vi "Four 64 bit to 256 bit pack.vi"(6 "Flush?":bool, 8 "Input Valid":bool, 11 "Input Data":u64) -> (0 "Output Valid":bool, 3 "Output Data":T1)   [LabVIEW 2011]
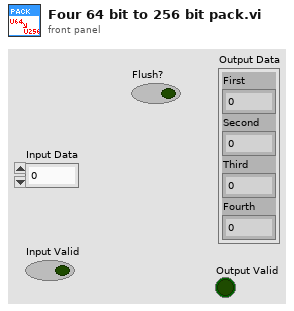
[diagram p1: front panel]
types:
  T1 = cluster{"First":u64, "Second":u64, "Third":u64, "Fourth":u64}
  T2 = cluster{"[0]":u64, "[1]":u64, "[2]":u64, "[3]":u64}
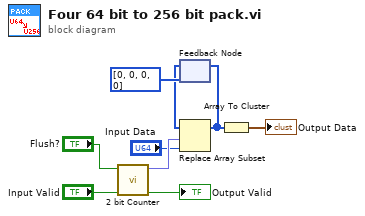
[diagram p0: block diagram]
diagram:
  n1 = call "2 bit Counter.vi"("Increment?"="Input Valid", "Reset?"="Flush?") -> ("Phase Match?"=→"Output Valid":bool, "counter value"=w7:fxp<+,2,2>)  [unwired: 8 in]
  n2 = feedback #1(u64[] [0, 0, 0, 0]) -> (w8:u64[])
  n3 = Replace Array Subset(array=w8, new element="Input Data", index=w7) -> (w3:u64[])
  n4 = feedback-in #1(w3) -> ()
  n5 = Array To Cluster(array=w3) -> (cluster=→"Output Data":T2)
